vi "Offset Point For Picture Control.vi"(10 "Point 2":T1, 11 "Point 1":T1) -> (3 "Offset Point":cluster{"horizontal":i16, "vertical":i16})   [LabVIEW 2015]
uses:
  Application Specific/Controls/Point 2D.ctl
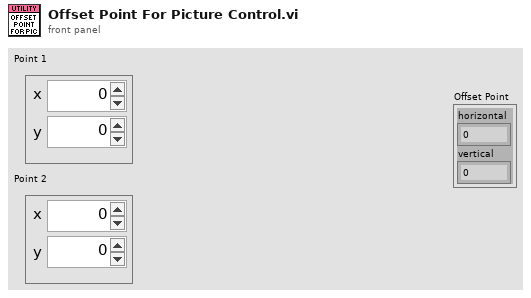
[diagram p1: front panel]
types:
  T1 = typedef "Point 2D.ctl" = cluster{"x":dbl, "y":dbl}
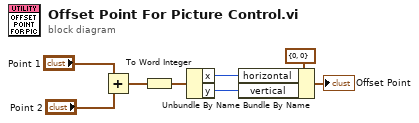
[diagram p0: block diagram]
diagram:
  n1 = Add(x="Point 1", y="Point 2") -> (x+y=w4:T1)
  n2 = To Word Integer(number=w4) -> (16bit integer=w3:cluster{"x":i16, "y":i16})
  n3 = Unbundle By Name(w3) -> ("x"=w2:i16, "y"=w1:i16)
  n4 = Bundle By Name(cluster=cluster{"horizontal":i16, "vertical":i16} {"horizontal"=0, "vertical"=0} ("pixel center"), "horizontal"=w2, "vertical"=w1) -> (→"Offset Point":cluster{"horizontal":i16, "vertical":i16})
